vi "MFC Test.vi"() -> ()   [LabVIEW 2014]
uses:
  <vilib>/rvi/interface/nirviOpenFPGA/nirviOpenFPGA.xnode
  <vilib>/rvi/interface/nirviReadWriteControl/nirviReadWriteControl.xnode
  <vilib>/rvi/interface/nirviCloseFPGA/nirviCloseFPGA.xnode
  FPGA main v05.vi
  NiFpgaLv.dll
  <vilib>/Utility/error.llb/Error Cluster From Error Code.vi
  <vilib>/rvi/interface/Simulation/niFpgaSimulationCallBeginRW.vi
  <vilib>/rvi/errors/niLvFpgaAdjustHostInterfaceError.vi
  <vilib>/FPGAPlugInAG/Dynamic/niLvFpga_Close_Dynamic.vi
panel:
  out "In Array 2":fxp<+/-,24,9>[](array[numeric])
  out "M7P4 string":string
  out "MFC M7P4":u8[](array[numeric])
  out "MFC M7P4 string":string
  in  "Out Array 3":u8[](array[numeric])=[66, 48, 48, 48, 48, 48, 13, 67, 48, 48, 48, 48, 48, 13, 73, 48, 48, 48, 48, 48, 13, 74, 48, 48, 48, 48, 48, 13, 75, 48, 48, 48, 48, 48, 13]
  out "MFC M8P1 string":string
  out "M8P1 string":string
  out "MFC M8P1":u8[](array[numeric])
  in  "stop":bool
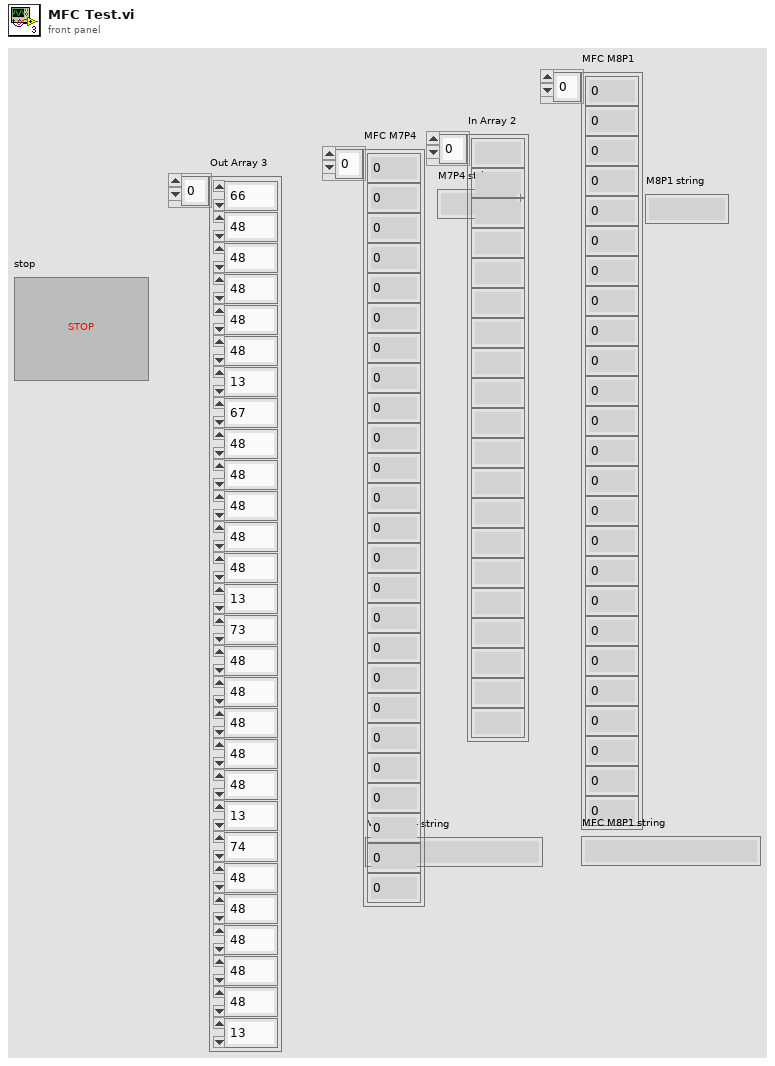
[diagram p1: front panel]
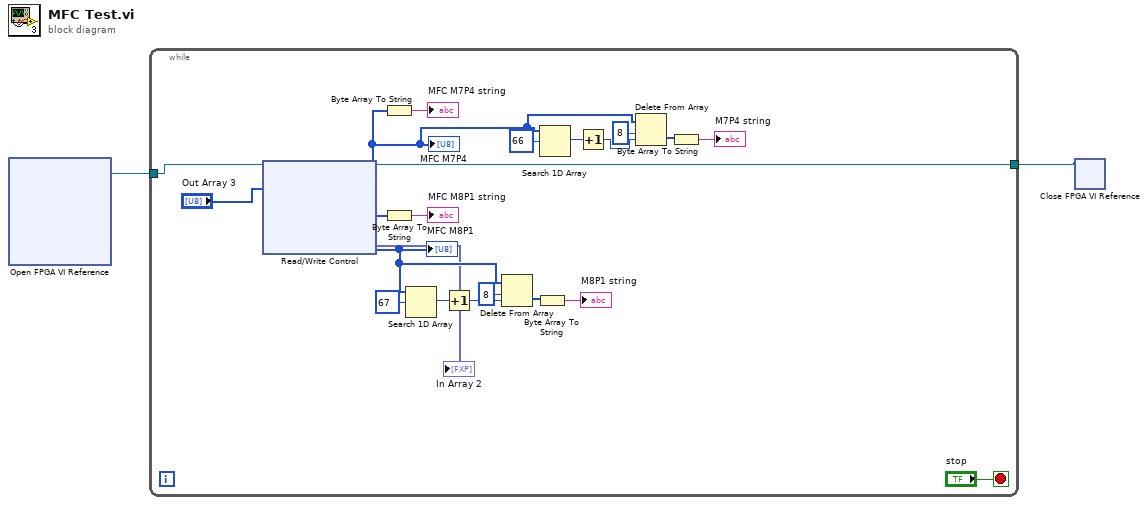
[diagram p0: block diagram]
diagram:
  n1 = xnode "Open FPGA VI Reference"() -> ("FPGA VI Reference Out"=w2:refnum<k20>)  [unwired: 2 in, 1 out]
  n2 = while {
    tunnel: w2 -> [w23]
    tunnel: [w22] -> w1
    stop <- "stop" stop-if-true
    n3 = xnode "Read/Write Control"("FPGA VI Reference In"=w23, "Out Array 2"="Out Array 3") -> ("FPGA VI Reference Out"=w22:refnum<k20>, "MFC HC out"=w5:u8[], "MFC AirC1 out"=w4:u8[], "In Array 2"=→"In Array 2":fxp<+/-,24,9>[])  [unwired: 1 in, 1 out]
    "MFC M8P1" <- w4
    "MFC M7P4" <- w5
    n4 = Byte Array To String(unsigned byte array=w5) -> (string=→"MFC M7P4 string":string)
    n5 = Byte Array To String(unsigned byte array=w4) -> (string=→"MFC M8P1 string":string)
    n6 = Search 1D Array(1D array=w4, element=u8 67) -> (index of element=w18:i32)  [unwired: 1 in]
    n7 = Increment(x=w18) -> (x+1=w17:i32)
    n8 = Delete From Array(array=w4, length=8, index=w17) -> (deleted portion=w16:u8[])  [unwired: 1 out]
    n9 = Byte Array To String(unsigned byte array=w16) -> (string=→"M8P1 string":string)
    n10 = Search 1D Array(1D array=w5, element=u8 66) -> (index of element=w8:i32)  [unwired: 1 in]
    n11 = Increment(x=w8) -> (x+1=w9:i32)
    n12 = Delete From Array(array=w5, length=8, index=w9) -> (deleted portion=w10:u8[])  [unwired: 1 out]
    n13 = Byte Array To String(unsigned byte array=w10) -> (string=→"M7P4 string":string)
  }
  n14 = xnode "Close FPGA VI Reference"("FPGA VI Reference In"=w1) -> ()  [unwired: 1 in, 1 out]
